vi "hidSPD Check Status.vi"(8 "error in (no error)":errorcluster, 11 "deviceInfo in":string) -> (0 "error out":errorcluster, 2 "available":bool, 3 "deviceInfo out":string)   [LabVIEW 2018, in "hidSPDLibForLabView.lvlib"]
uses:
  hidSPDLibForLabView.lvlib
  hidSPD DLL files/libSPD.dll
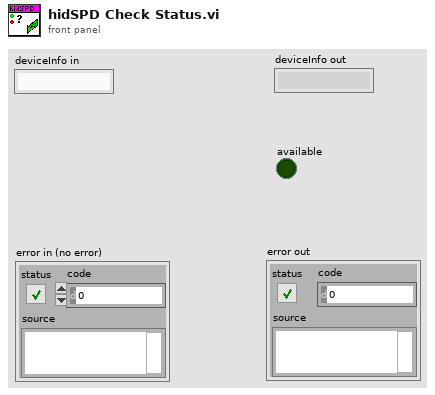
[diagram p1: front panel]
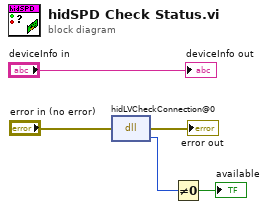
[diagram p0: block diagram]
diagram:
  n1 = dll-call lib="F:/NextCloud/SPD stand/Automative SPD Measurements/v 1.0.0/Instruments/SPD HID Interface/hidSPD DLL files/libSPD.dll" fn="hidLVCheckConnection@0"(error in="error in (no error)") -> (error out=→"error out":errorcluster, "return type"=w5:i32)  [unwired: 2 in, 1 out]
  n2 = Not Equal To 0?(x=w5) -> (x != 0?=→"available":bool)
  "deviceInfo out" <- "deviceInfo in"
